vi "ohsp Single Measurement.vi"() -> ()   [LabVIEW 2012]
doc: "This VI will take a single measurement in the units selected."
panel:
  in  "Units (0: Gram)":u16(ring) items=["Gram (g)", "Ounce (oz)", "Troy Ounce (oz t)", "Pennyweight (dwt)", "Parts Counting (PC)", "Pound (lb)", "Newton (N)", "Kilogram (kg)", "lb or oz on some models", "Percent (%)"]
  in  "Serial Configuration":T1={"Baud Rate (2400)"=2400, "Flow Control (2: RTS/CTS)"=2, "Parity (0: None)"=0, "Data Bits (7)"=7} {"Data Bits (7)" items=["7"=7, "8"=8]; "Parity (0: None)" items=["None", "Odd", "Even"]; "Flow Control (2: RTS/CTS)" items=["None", "XON/XOFF", "RTS/CTS"]; "Baud Rate (2400)" items=["600"=600, "1200"=1200, "2400"=2400, "4800"=4800, "9600"=9600, "19200"=19200]}
  in  "VISA resource name":refnum<visa-resource-name>="COM1"
  out "Stable?":bool
  out "Units":string
  out "Weight Value":dbl format="%.2g"
  # "© 2004 National Instruments.  All Rights Reserved."
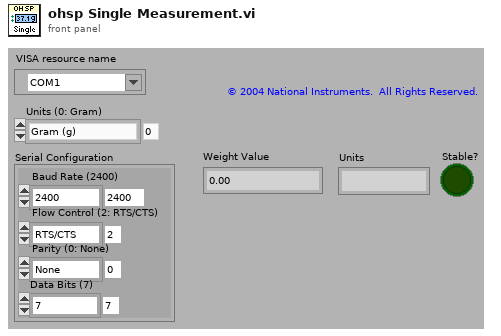
[diagram p1: front panel]
types:
  T1 = cluster{"Baud Rate (2400)":u32, "Flow Control (2: RTS/CTS)":u16, "Parity (0: None)":u16, "Data Bits (7)":u16}
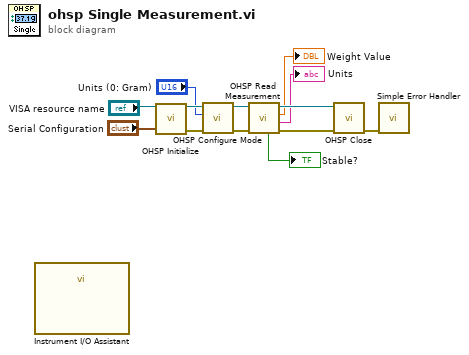
[diagram p0: block diagram]
diagram:
  n1 = call "Instrument I/O Assistant"() -> ()  [unwired: 28 in]
  n2 = call <instrlib>:"OHSP Initialize.vi"("VISA resource name"="VISA resource name", "Serial Configuration"="Serial Configuration") -> ("VISA resource name out"=w12:refnum<visa-resource-name>, "error out"=w13:errorcluster)  [unwired: 12 in]
  n3 = call <instrlib>:"OHSP Configure Mode.vi"("error in (no error)"=w13, "Units (0: Gram)"="Units (0: Gram)", "VISA resource name"=w12) -> ("error out"=w11:errorcluster, "VISA resource name out"=w10:refnum<visa-resource-name>)  [unwired: 7 in]
  n4 = call <instrlib>:"OHSP Read Measurement.vi"("error in (no error)"=w11, "VISA resource name"=w10) -> ("error out"=w9:errorcluster, "Units"=→"Units":string, "Weight Value"=→"Weight Value":dbl, "VISA resource name out"=w8:refnum<visa-resource-name>, "Stable?"=→"Stable?":bool)  [unwired: 5 in]
  n5 = call <instrlib>:"OHSP Close.vi"("error in (no error)"=w9, "VISA resource name"=w8) -> ("error out"=w4:errorcluster)  [unwired: 8 in]
  n6 = call <vilib>:"Simple Error Handler.vi"("error in (no error)"=w4) -> ()  [unwired: 4 in, 5 out]
